vi "Do.vi"(8 "error in (no error)":errorcluster, 10 "Actor in":refnum<class "Actor.lvclass">, 11 "Write Blink Msg":refnum<class "Write Blink Msg.lvclass">) -> (0 "error out":errorcluster, 2 "Actor out":refnum<class "Actor.lvclass">)   [LabVIEW 2014, in "Display Panel.lvlib" / "Write Blink Msg.lvclass"]
doc: "This VI delivers the message to the actor by calling the appropriate method(s) on the actor."
uses:
  Write Blink Msg.lvclass
  <vilib>/ActorFramework/Actor/Actor.lvclass
  Power Meter Display/Power Meter Display.lvclass
  Write Blink Msg.lvclass/Write Blink Msg.ctl
  Abstract Display/Abstract Display.lvclass/Abstract Display.ctl
  Abstract Display/Abstract Display.lvclass
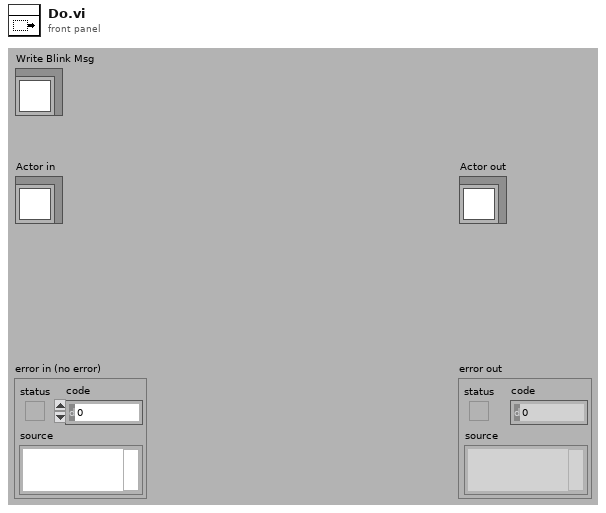
[diagram p1: front panel]
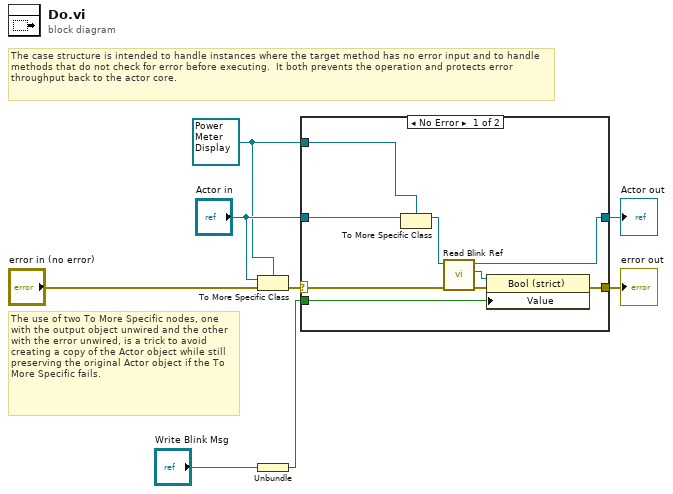
[diagram p0: block diagram]
diagram:
  w2 = refnum<class "Power Meter Display.lvclass"> refnum ("Actor in")
  # "The use of two To More Specific nodes, one with the output object unwired and the other with the error unwired, is a trick to avoid creating a copy of the Actor object while still preserving the original Actor object if the To More Specific fails."
  # "The case structure is intended to handle instances where the target method has no error input and to handle methods that do not check for error before executing.  It both prevents the operation and protects error throughput back to the actor core."
  n1 = To More Specific Class(target class=w2, reference="Actor in", error in="error in (no error)") -> (error out=w6:errorcluster)  [unwired: 1 out]
  n2 = Unbundle("Write Blink Msg") -> (w1:bool)
  n3 = case shown="No Error" w6 {
    selector: w6 -> [w11 w19]
    tunnel: [w9 w19] -> w5
    tunnel: [w12 w18] -> w4
    tunnel: "Actor in" -> [w17 w18]
    tunnel: w2 -> [w16 _]
    tunnel: w1 -> [w13 _]
    frame No Error {
      n4 = To More Specific Class(target class=w16, reference=w17) -> (specific class reference=w15:refnum<class "Power Meter Display.lvclass">)  [unwired: 1 in, 1 out]
      n5 = call "Read Blink Ref.vi"("error in (no error)"=w11, "Abstract Display in"=w15) -> ("error out"=w10:errorcluster, "Blink? Ref"=w14:refnum<vi>, "Abstract Display out"=w12:refnum<class "Power Meter Display.lvclass">)  [unwired: 7 in]
      n6 = property class="Bool (strict)"(reference=w14, error in=w10, "Value"=w13) -> (error out=w9:errorcluster)  [unwired: 1 out]
    }
    frame Error {
      # "If type check fails, pass the original object out again."
    }
  }
  "error out" <- w5
  "Actor out" <- w4
